vi "get_parametrisation_angles.vi"(8 "error in (no error)":errorcluster, 11 "TrajectoryDL110420DoubleCircle in":refnum<class "TrajectoryDL110420DoubleCircle.lvclass">) -> (0 "error out":errorcluster, 2 "angles":dbl[](array[numeric]), 3 "TrajectoryDL110420DoubleCircle out":refnum<class "TrajectoryDL110420DoubleCircle.lvclass">)   [LabVIEW 2010, in "TrajectoryDL110420DoubleCircle.lvclass"]
uses:
  TrajectoryDL110420DoubleCircle.lvclass
  TrajectoryDL110420DoubleCircle.lvclass/TrajectoryDL110420DoubleCircle.ctl
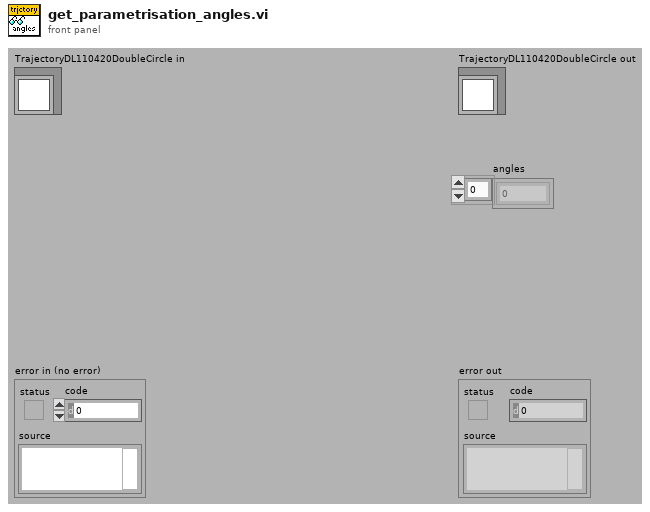
[diagram p1: front panel]
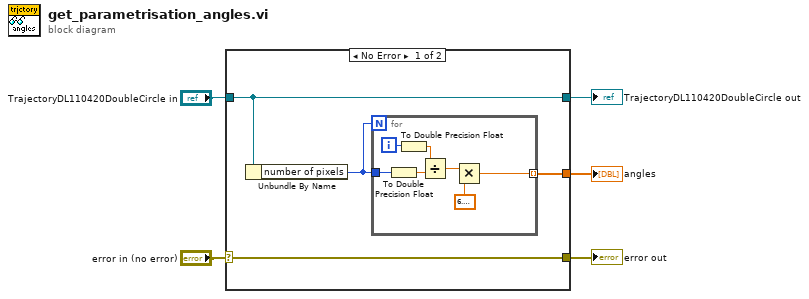
[diagram p0: block diagram]
diagram:
  n1 = case shown="No Error" "error in (no error)" {
    selector: "error in (no error)" -> [w9 w18]
    tunnel: [w9 w18] -> w4
    tunnel: [w8 w17] -> w2
    tunnel: "TrajectoryDL110420DoubleCircle in" -> [w8 w17]
    tunnel: [w7 _] -> w1
    frame No Error {
      n2 = Unbundle By Name(w8) -> ("number of pixels"=w6:i32)
      n3 = for {
        N: w6 -> [_]
        tunnel: w6 -> [w16]
        tunnel: [w10] -> w7 mode=indexing
        i -> [w13]
        n4 = To Double Precision Float(number=w16) -> (double precision float=w14:dbl)
        n5 = To Double Precision Float(number=w13) -> (double precision float=w12:dbl)
        n6 = Divide(x=w12, y=w14) -> (x/y=w11:dbl)
        n7 = Multiply(x=w11, y=6.283185307179586) -> (x*y=w10:dbl)
      }
    }
    frame Error {
    }
  }
  "error out" <- w4
  "TrajectoryDL110420DoubleCircle out" <- w2
  "angles" <- w1
